vi "ClearData.vi"(8 "error in (no error)":errorcluster, 10 "Task":string, 11 "DAQ_Module in":refnum<class "DAQ_Module.lvclass">) -> (0 "error out":errorcluster, 3 "DAQ_Module out":refnum<class "DAQ_Module.lvclass">)   [LabVIEW 2025, in "DAQ_Module.lvlib" / "DAQ_Module.lvclass"]
uses:
  DAQ_Module.lvclass
  DAQ_Module.lvclass/DAQ_Module.ctl
  DAQ_Abstr/Task_Abstr/Task_Abstr Messages/ClearDataContainer Msg/ClearDataContainer Msg.lvclass
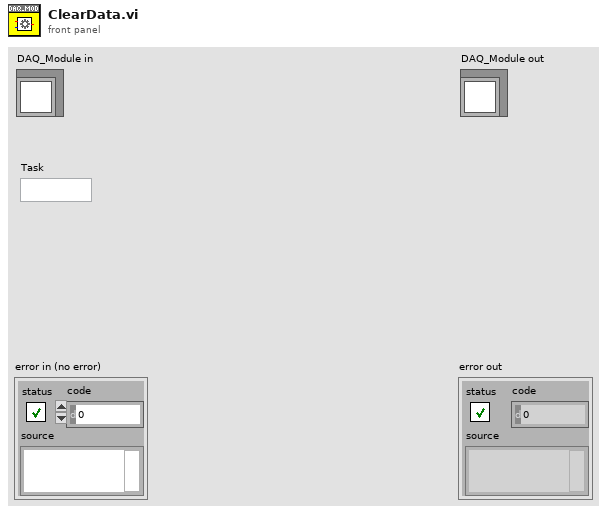
[diagram p1: front panel]
types:
  T1 = map{string, refnum<class "Message Enqueuer.lvclass">}
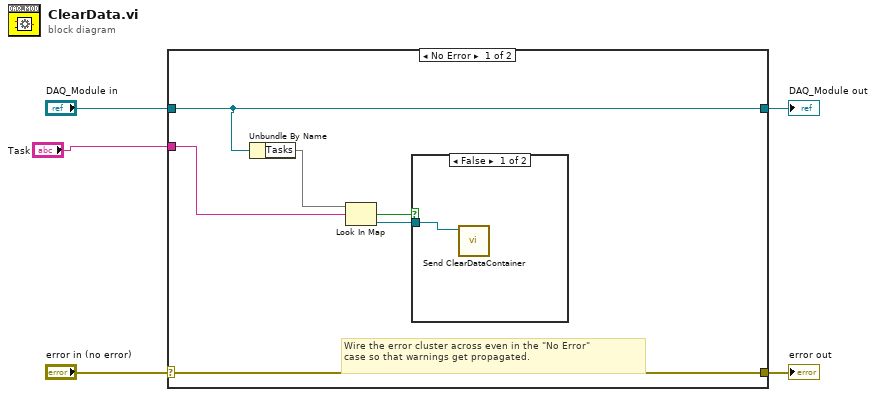
[diagram p0: block diagram]
diagram:
  n1 = case shown="No Error" "error in (no error)" {
    selector: "error in (no error)" -> [w11 w14]
    tunnel: [w11 w14] -> w4
    tunnel: [w7 w13] -> w2
    tunnel: "DAQ_Module in" -> [w7 w13]
    tunnel: "Task" -> [w6 _]
    frame No Error {
      # "Wire the error cluster across even in the \"No Error\"\ncase so that warnings get propagated."
      n2 = Unbundle By Name(w7) -> ("Tasks"=w10:T1)
      n3 = Look In Map(map=w10, key=w6) -> (key not found?=w8:bool, value=w9:refnum<class "Message Enqueuer.lvclass">)  [unwired: 1 in]
      n4 = case shown="False" w8 {
        tunnel: w9 -> [w12 _]
        frame False {
          n5 = call "Send ClearDataContainer.vi"("Message Enqueuer"=w12) -> ()  [unwired: 9 in, 2 out]
        }
        frame True {
        }
      }
    }
    frame Error {
    }
  }
  "error out" <- w4
  "DAQ_Module out" <- w2
